vi "closeArduinoNew.vi"   [LabVIEW 2012]
uses:
  GlobalArduinoNew.vi
  <vilib>/LabVIEW Interface for Arduino/LabVIEW Interface for Arduino.lvlib
types:
  T1 = typedef "Semaphore RefNum" = refnum<k1>
  T2 = typedef "LabVIEW Interface for Arduino.lvlib/Arduino Resource.ctl" = cluster{"VISA resource":refnum<visa-resource-name>, "Board Type":T3, "Connection Type":enum8{"USB / Serial"}, "Bytes Per Packet (15)":u8}
  T3 = typedef "LabVIEW Interface for Arduino.lvlib/Board Type.ctl" = enum16{"Uno", "Dimuelanove w/Atmega 328", "Mega 2560"}
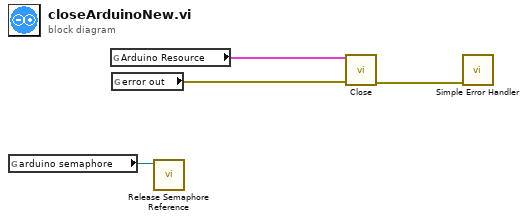
[diagram p0: block diagram]
diagram:
  n1 = global read "GlobalArduinoNew.vi" "arduino semaphore"() -> (w1:T1)
  n2 = global read "GlobalArduinoNew.vi" "Arduino Resource"() -> (w3:T2)
  n3 = global read "GlobalArduinoNew.vi" "error out"() -> (w2:errorcluster)
  n4 = call <vilib>:"Release Semaphore Reference.vi"("semaphore"=w1) -> ()  [unwired: 9 in, 2 out]
  n5 = call <vilib>:"Close.vi"("Arduino Resource"=w3, "error in"=w2) -> ("error out"=w4:errorcluster)  [unwired: 13 in]
  n6 = call <vilib>:"Simple Error Handler.vi"("error in (no error)"=w4) -> ()  [unwired: 4 in, 5 out]
